vi "ACT_LabVIEW3_Task1_Team072.vi"() -> ()   [LabVIEW 2016]
panel:
  out "Iterations":dbl
  in  "Upper Limit":dbl
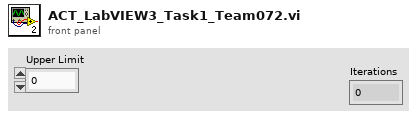
[diagram p1: front panel]
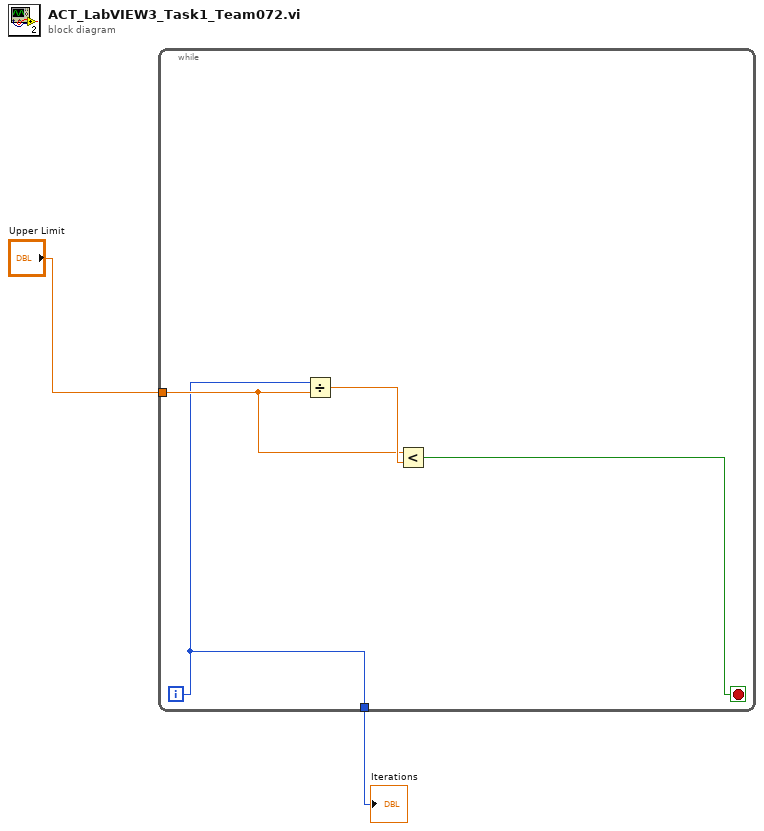
[diagram p0: block diagram]
diagram:
  n1 = while {
    tunnel: "Upper Limit" -> [w4]
    tunnel: [w3] -> w1
    i -> [w3]
    stop <- w6 stop-if-true
    n2 = Divide(x=w3, y=w4) -> (x/y=w5:dbl)
    n3 = Less?(x=w4, y=w5) -> (x < y?=w6:bool)
  }
  "Iterations" <- w1
